vi "resetDAQDevice.vi"(8 "error in (no error)":errorcluster, 11 "device in":tag) -> (0 "error out":errorcluster)   [LabVIEW 2015]
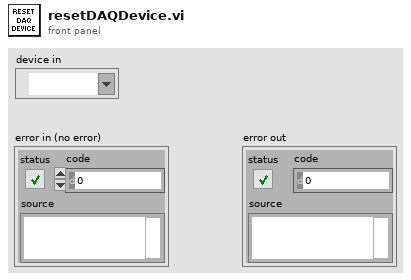
[diagram p1: front panel]
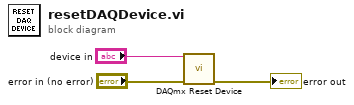
[diagram p0: block diagram]
diagram:
  n1 = call <vilib>:"DAQmx Reset Device.vi"("device in"="device in", "error in"="error in (no error)") -> ("error out"=→"error out":errorcluster)  [unwired: 13 in]
